vi "power measure.vi"(9 "input valid":bool, 10 "sample":T1) -> (1 "output valid":bool, 2 "output":fxp<+,38,6>)   [LabVIEW 2020]
uses:
  <vilib>/rvi/FXPMathLib/FxpInterpret/XNode/nifxpmath_Interpret.xnode
types:
  T1 = cluster{"Real":fxp<+/-,16,3>, "Imag":fxp<+/-,16,3>}
  T2 = cluster{"Real":fxp<+/-,25,25>, "Imag":fxp<+/-,25,25>}
  T3 = cluster{"Real":fxp<+/-,18,18>, "Imag":fxp<+/-,18,18>}
  T4 = cluster{"Real":fxp<+/-,48,48>, "Imag":fxp<+/-,48,48>}
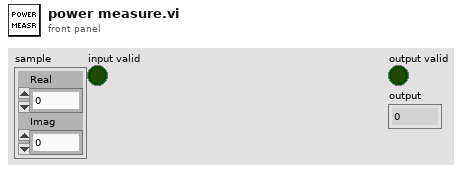
[diagram p1: front panel]
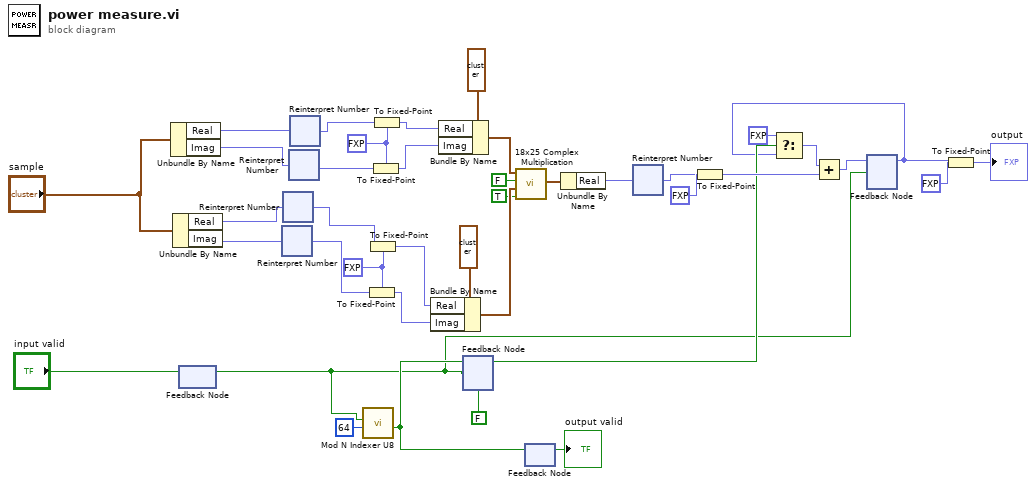
[diagram p0: block diagram]
diagram:
  w23 = fxp<+/-,25,25> 0.0 ("fixed-point type")
  w28 = fxp<+/-,18,18> 0.0 ("fixed-point type")
  n1 = Unbundle By Name("sample") -> ("Real"=w38:fxp<+/-,16,3>, "Imag"=w37:fxp<+/-,16,3>)
  n2 = Unbundle By Name("sample") -> ("Real"=w36:fxp<+/-,16,3>, "Imag"=w35:fxp<+/-,16,3>)
  n3 = feedback-in #1("input valid") -> ()
  n4 = feedback #1() -> (w4:bool)  [unwired: 1 in]
  n5 = xnode "Reinterpret Number"("x"=w35) -> ("y"=w21:fxp<+/-,16,16>)
  n6 = xnode "Reinterpret Number"("x"=w36) -> ("y"=w22:fxp<+/-,16,16>)
  n7 = xnode "Reinterpret Number"("x"=w37) -> ("y"=w24:fxp<+/-,16,16>)
  n8 = xnode "Reinterpret Number"("x"=w38) -> ("y"=w25:fxp<+/-,16,16>)
  n9 = call "Mod N Indexer U8.vi"("N"=u8 64, "enable"=w4) -> ("wrap back"=w6:bool)  [unwired: 8 in, 1 out]
  n10 = To Fixed-Point(fixed-point type=w23, number=w21) -> (fixed-point=w19:fxp<+/-,25,25>)
  n11 = To Fixed-Point(fixed-point type=w23, number=w22) -> (fixed-point=w20:fxp<+/-,25,25>)
  n12 = To Fixed-Point(fixed-point type=w28, number=w24) -> (fixed-point=w26:fxp<+/-,18,18>)
  n13 = To Fixed-Point(fixed-point type=w28, number=w25) -> (fixed-point=w27:fxp<+/-,18,18>)
  n14 = Bundle By Name(cluster=T2 {"Real"=0.0, "Imag"=0.0} ("Complex"), "Real"=w20, "Imag"=w19) -> (w31:T2)
  n15 = Bundle By Name(cluster=T3 {"Real"=0.0, "Imag"=0.0} ("Complex"), "Real"=w27, "Imag"=w26) -> (w32:T3)
  n16 = feedback-in #2(w6, w4) -> ()
  n17 = feedback #2(FALSE ("wrap back")) -> (w9:bool)
  n18 = call "18x25 Complex Multiplication.vi"("conjugate B"=TRUE, "B"=w31, "conjugate A"=FALSE, "A"=w32) -> ("product"=w16:T4)  [unwired: 7 in]
  n19 = feedback #3() -> (→"output valid":bool)  [unwired: 1 in]
  n20 = feedback-in #3(w6) -> ()
  n21 = Unbundle By Name(w16) -> ("Real"=w15:fxp<+/-,48,48>)
  n22 = xnode "Reinterpret Number"("x"=w15) -> ("y"=w13:fxp<+/-,48,22>)
  n23 = To Fixed-Point(fixed-point type=fxp<+,32,6> 0.0, number=w13) -> (fixed-point=w12:fxp<+,32,6>)
  n24 = feedback #4() -> (w2:fxp<+,38,12>)  [unwired: 1 in]
  n25 = Select(t=fxp<+,32,6> 0.0 ("fixed-point type"), s=w9, f=w2) -> (s? t:f=w11:fxp<+,38,12>)
  n26 = Add(x=w11, y=w12) -> (x+y=w8:fxp<+,38,12>)
  n27 = feedback-in #4(w8, w4) -> ()
  n28 = To Fixed-Point(fixed-point type=fxp<+,38,6> 0.0, number=w2) -> (fixed-point=→"output":fxp<+,38,6>)
